vi "ReadCaseMonitor__slk_mt.vi"(8 "error in (no error)":errorcluster, 11 "refnum in":T1) -> (0 "error out":errorcluster, 2 "case monitor configure":T2, 3 "refnum out":T1)   [LabVIEW 2015]
doc: "Gets configure datum of Case Monitor.\n\n<b>[Case Monitor]</b>\nParent Symbol = \"-\""
uses:
  TypeDef/TypeDef_CaseMonitorConfigure__slk_mt.ctl
  <vilib>/Utility/config.llb/Config Data RefNum.ctl
  <vilib>/Utility/config.llb/Read Key (String).vi
  <vilib>/Utility/config.llb/NI_LVConfig.lvlib
panel:
  # "ReadCaseMonitor__slk_mt.vi\nGets configure datum of Case Monitor.\n\nNOTICE -- YOU MUST LEAVE THIS NOTICE IN PLACE.\n\nCopyright (c) 2011, LIANG LIU Shawn.Liu.cn@gmail.com\nAll rights reserved.\n\nRedistribution and use in source and binary forms, with or without modification, are permitted provided that the following conditions are met:\n-Redistributions of source code must retain the above copyright notice, this list of conditions and the following disclaimer.\n-Redistributions in binary form must reproduce the above copyright notice, this list of conditions and the following disclaimer in the documentation and/or other materials provided with the distribution.\n-Neither the name of the eLp nor the names of its contributors may be used to endorse or promote products derived from this software without specific prior written permission.\n\nTHIS SOFTWARE IS PROVIDED BY THE COPYRIGHT HOLDERS AND CONTRIBUTORS \"AS IS\" AND ANY EXPRESS OR IMPLIED WARRANTIES, INCLUDING, BUT NOT LIMITED TO, THE IMPLIED WARRANTIES OF MERCHANTABILITY AND FITNESS FOR A PARTICULAR PURPOSE ARE DISCLAIMED. IN NO EVENT SHALL THE COPYRIGHT HOLDER OR CONTRIBUTORS BE LIABLE FOR ANY DIRECT, INDIRECT, INCIDENTAL, SPECIAL, EXEMPLARY, OR CONSEQUENTIAL DAMAGES (INCLUDING, BUT NOT LIMITED TO, PROCUREMENT OF SUBSTITUTE GOODS OR SERVICES; LOSS OF USE, DATA, OR PROFITS; OR BUSINESS INTERRUPTION) HOWEVER CAUSED AND ON ANY THEORY OF LIABILITY, WHETHER IN CONTRACT, STRICT LIABILITY, OR TORT (INCLUDING NEGLIGENCE OR OTHERWISE) ARISING IN ANY WAY OUT OF THE USE OF THIS SOFTWARE, EVEN IF ADVISED OF THE POSSIBILITY OF SUCH DAMAGE."
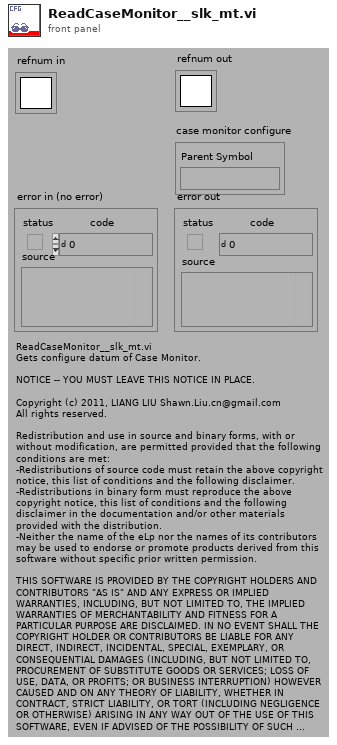
[diagram p1: front panel]
types:
  T1 = typedef "NI_LVConfig.lvlib/Config Data RefNum.ctl" = refnum<k1>
  T2 = typedef "TypeDef_CaseMonitorConfigure__slk_mt.ctl" = cluster{"Parent Symbol":string}
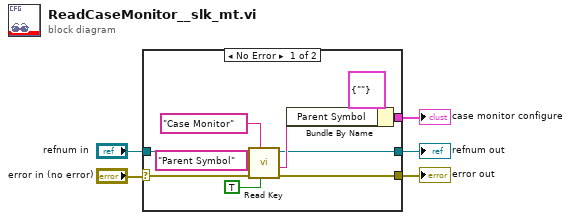
[diagram p0: block diagram]
diagram:
  n1 = case shown="No Error" "error in (no error)" {
    selector: "error in (no error)" -> [w12 w17]
    tunnel: "refnum in" -> [w15 w16]
    tunnel: [w7 w16] -> w4
    tunnel: [w11 _] -> w1
    tunnel: [w8 w17] -> w2
    frame No Error {
      n2 = call-poly <vilib>:"Read Key.vi"("read raw string? (F)"=TRUE, "section"="Case Monitor", "error in (no error)"=w12, "key"="Parent Symbol", "refnum"=w15) -> ("error out"=w8:errorcluster, "value"=w13:string, "refnum out"=w7:T1)  [unwired: 3 in, 1 out]
      n3 = Bundle By Name(cluster=T2 {"Parent Symbol"=""} ("Cae Monitor Configure"), "Parent Symbol"=w13) -> (w11:T2)
    }
    frame Error {
    }
  }
  "case monitor configure" <- w1
  "error out" <- w2
  "refnum out" <- w4
